vi "test_PV_String.vi"() -> ()   [LabVIEW 2013]
panel:
  out "data 6":string
  in  "Hexadecimal Input String":string
  out "Decimal value":i32
  out "data 5":i32
  out "data 4":variant
  out "data 3":dbl
  out "quality":u64
  out "Numeric":i32
  out "data":string[](array[string])
  out "data 2":string
  in  "stop":bool
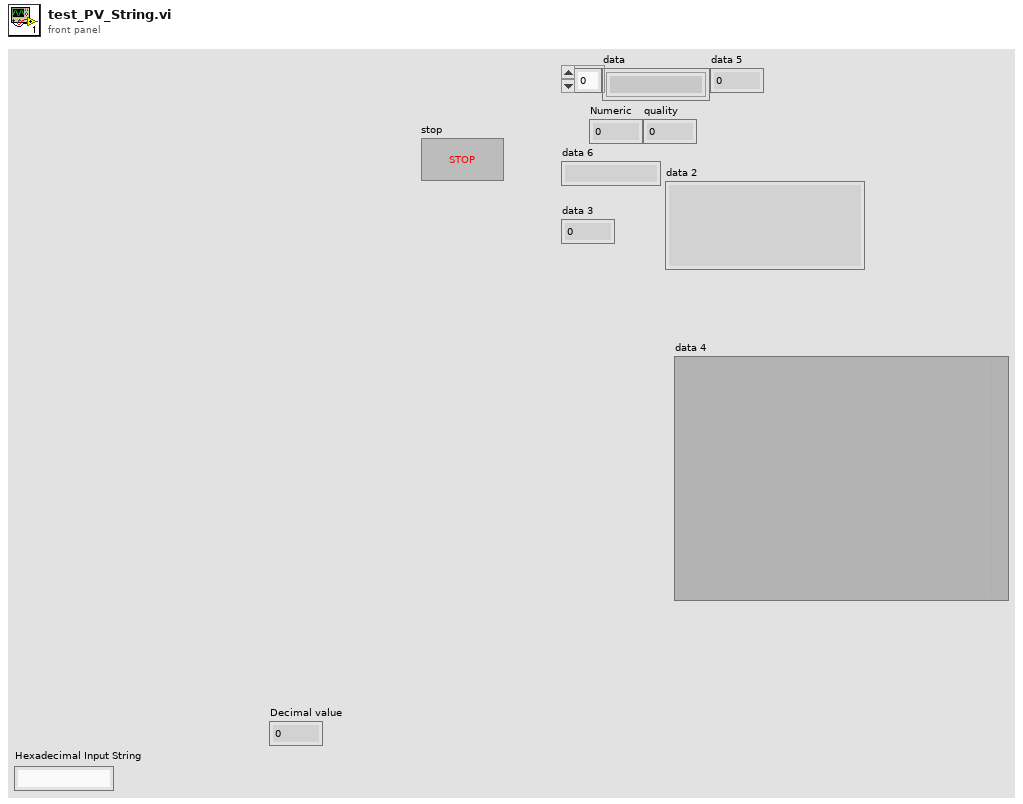
[diagram p1: front panel]
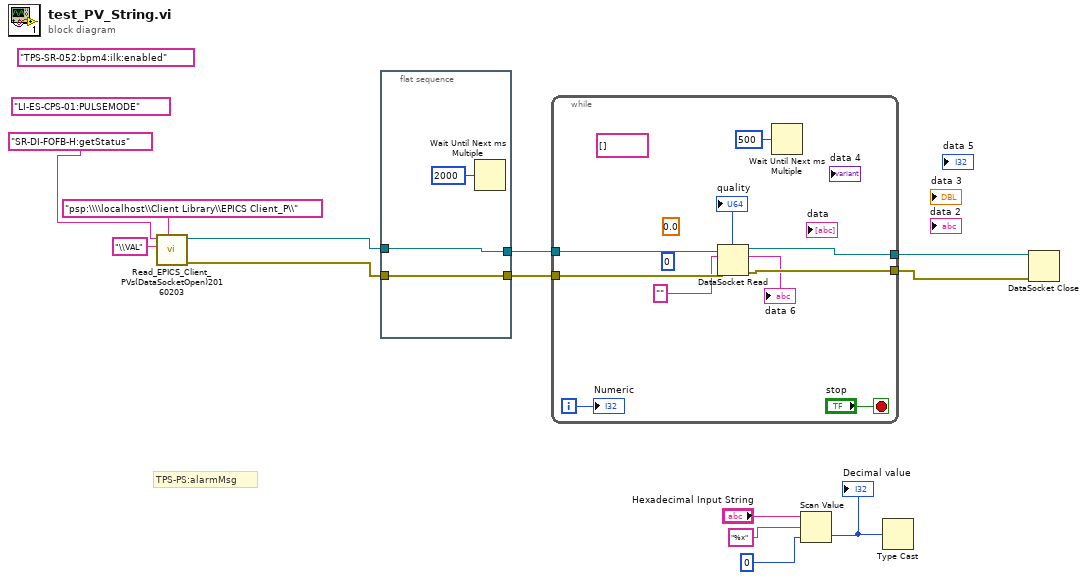
[diagram p0: block diagram]
diagram:
  (unwired) "TPS-SR-052:bpm4:ilk:enabled"
  (unwired) "LI-ES-CPS-01:PULSEMODE"
  # "TPS-PS:alarmMsg"
  n1 = call "Read_EPICS_Client_PVs(DataSocketOpen)20160203.vi"("LLB"="psp:\\\\localhost\\Client Library\\EPICS Client_P\\", "field"="\\VAL", "PV name"="SR-DI-FOFB-H:getStatus") -> ("error out"=w5:errorcluster, "connection id"=w7:refnum<k13>)  [unwired: 7 in]
  n2 = flat-sequence {
    tunnel: [w16] -> w8
    tunnel: w7 -> [w16]
    tunnel: [w15] -> w6
    tunnel: w5 -> [w15]
    frame #0 {
      n3 = Wait Until Next ms Multiple(millisecond multiple=u32 2000) -> ()  [unwired: 1 out]
    }
  }
  n4 = while {
    tunnel: w8 -> [w26]
    tunnel: [w25] -> w11
    tunnel: [w24] -> w10
    tunnel: w6 -> [w23]
    i -> [w20]
    stop <- "stop" stop-if-true
    (unwired) string[] []
    (unwired) 0
    (unwired) 0.0
    n5 = DataSocket Read(8:w23, 10:"", 11:w26) -> (0:w24:errorcluster, 2:→"data 6":string, 3:w25:refnum<k13>, 5:→"quality":u64)  [unwired: 2 in, 3 out]
    n6 = Wait Until Next ms Multiple(millisecond multiple=u32 500) -> ()  [unwired: 1 out]
    "Numeric" <- w20
  }
  n7 = Scan Value(string="Hexadecimal Input String", format string="%x", default (0 dbl)=0 ("offset (0)")) -> (value=w4:i32)  [unwired: 1 out]
  "Decimal value" <- w4
  n8 = Type Cast(x=w4) -> ()  [unwired: 1 in, 1 out]
  n9 = DataSocket Close(8:w10, 11:w11) -> ()  [unwired: 1 in, 2 out]
